vi "UpdateMarks(SubVI).vi"(9 "MarksEarned":variant, 10 "QuestionsNo_Ordered":string, 11 "connection reference":T1) -> ()   [LabVIEW 2013]
uses:
  <vilib>/addons/database/Connection.llb/Conn ObjectReference.ctl
  FYP_LabviewGlobal(SubVI).vi
  <vilib>/addons/database/_DB Variant To Data/Database Variant To Data.xnode
  <vilib>/addons/database/NI_Database_API.lvlib
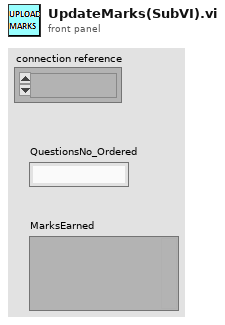
[diagram p1: front panel]
types:
  T1 = typedef "NI_Database_API.lvlib/Conn ObjectReference.ctl" = refnum<k1>
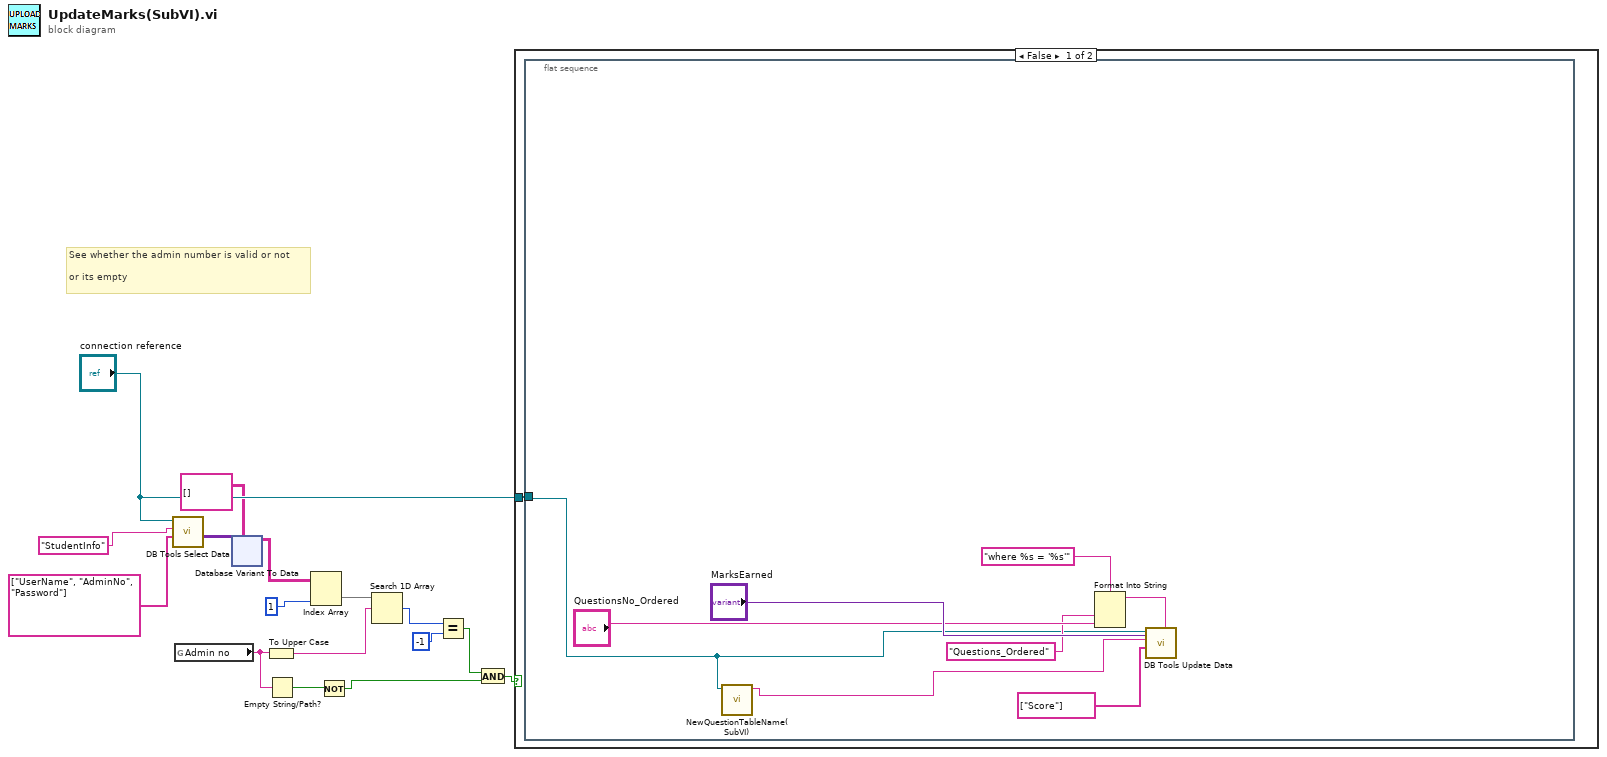
[diagram p0: block diagram]
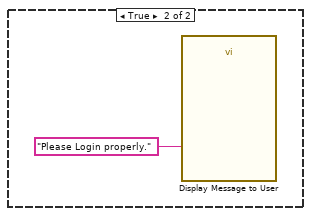
[diagram p2: hidden frame]
diagram:
  # "See whether the admin number is valid or not\n\nor its empty"
  n1 = call <vilib>:"DB Tools Select Data.vi"("columns"=string[] ["UserName", "AdminNo", "Password"], "table"="StudentInfo", "connection reference"="connection reference") -> ("data"=w13:variant[][])  [unwired: 3 in, 2 out]
  n2 = global read "FYP_LabviewGlobal(SubVI).vi" "Admin no"() -> (w3:string)
  n3 = xnode "Database Variant To Data"("database variant"=w13, "type"=string[][] []) -> ("data"=w11:string[][])  [unwired: 1 in, 1 out]
  n4 = To Upper Case(1:w3) -> (0:w8:string)
  n5 = Empty String/Path?(string/path=w3) -> (empty?=w4:bool)
  n6 = Index Array(array=w11, index (col)=1) -> (element=w9:string[])  [unwired: 1 in]
  n7 = Not(x=w4) -> (.not. x?=w2:bool)
  n8 = Search 1D Array(1D array=w9, element=w8) -> (index of element=w5:i32)  [unwired: 1 in]
  n9 = Equal?(x=w5, y=-1) -> (x = y?=w7:bool)
  n10 = And(x=w7, y=w2) -> (x .and. y?=w1:bool)
  n11 = case shown="False" w1 {
    tunnel: "connection reference" -> [w17 _]
    frame False {
      n12 = flat-sequence {
        tunnel: w17 -> [w18]
        frame #0 {
          n13 = call "NewQuestionTableName(SubVI).vi"("connection reference"=w18) -> ("String"=w19:string)  [unwired: 9 in, 1 out]
          n14 = Format Into String(format string="where %s = '%s'", "Questions_Ordered", "QuestionsNo_Ordered") -> (resulting string=w22:string)  [unwired: 2 in, 1 out]
          n15 = call <vilib>:"DB Tools Update Data.vi"("condition"=w22, "data"="MarksEarned", "columns"=string[] ["Score"], "table"=w19, "connection reference"=w18) -> ()  [unwired: 5 in, 2 out]
        }
      }
    }
    frame True {
      n16 = call "Display Message to User"("Message"="Please Login properly.") -> ()  [unwired: 9 in, 2 out]
    }
  }
